vi "Destroy User Event - Error.vi"(8 "error in (no error)":errorcluster, 11 "UE Error":refnum<user-event>) -> (0 "error out":errorcluster)   [LabVIEW 2017, in "User Events.lvlib"]
doc: "Destroy the user event, even if there is an incoming error."
uses:
  User Events.lvlib
  Error Handler/Controls/Error EventData.ctl
  Error Handler/Controls/Error Type.ctl
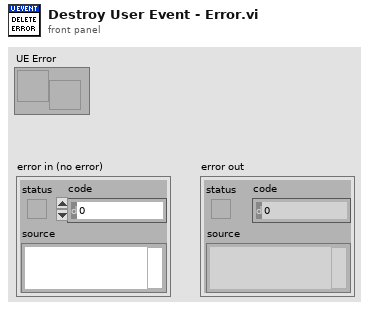
[diagram p1: front panel]
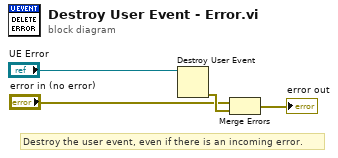
[diagram p0: block diagram]
diagram:
  # "Destroy the user event, even if there is an incoming error."
  n1 = Destroy User Event(user event="UE Error") -> (error out=w4:errorcluster)  [unwired: 1 in]
  n2 = Merge Errors("error in (no error)", w4) -> (→"error out":errorcluster)
